vi "main.vi"() -> ()   [LabVIEW 2020]
uses:
  Libreria propria Chroma63204A/chr63204A_Error_conversion.vi
panel:
  out "CURR":dbl
  out "VOLT":dbl
  out "Numeric":i32
  out "element":dbl
  out "x = y?":bool
  out "error out (no error) 2":errorcluster
  in  "timestep (s)":u32=1
  in  "Load from file":bool
  in  "Load Profile path":path=path "C:/Users/thoma/Desktop/Nuova cartella/Load profile.csv"
  out "error out (no error)":errorcluster
  in  "Save path":path=path "C:/Users/thoma/Desktop/main/log.csv"
  in  "Stop Button":bool
  in  "LOAD":bool
  in  "Set current (A)":dbl
  in  "error in (no error)":errorcluster
  in  "Chroma USB port":refnum<visa-resource-name>
  in  "Mode":u16(ring)=1 items=["Z", "CC", "CR", "CV", "CP", "CCD", "CRD", "BAT", "SWD", "OCP", "CCS", "CZ", "CVCC", "CRCC", "CVCR", "AUTO", "PROG", "UDW", "EXT"]
  out "LOAD_STATE":bool
  out "Current imposed":dbl
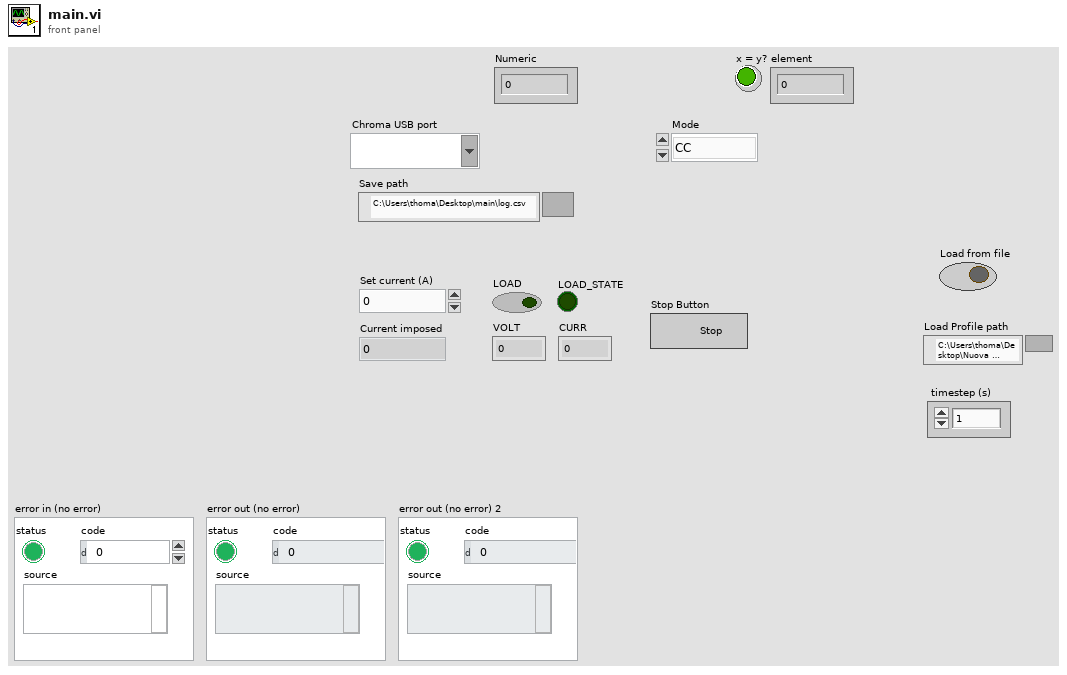
[diagram p1: front panel]
types:
  T1 = enum16{"open", "replace", "create", "open or create", "replace or create", "replace or create with confirmation"}
  T2 = enum8{"Enabled", "Disabled", "Disabled and Grayed Out"}
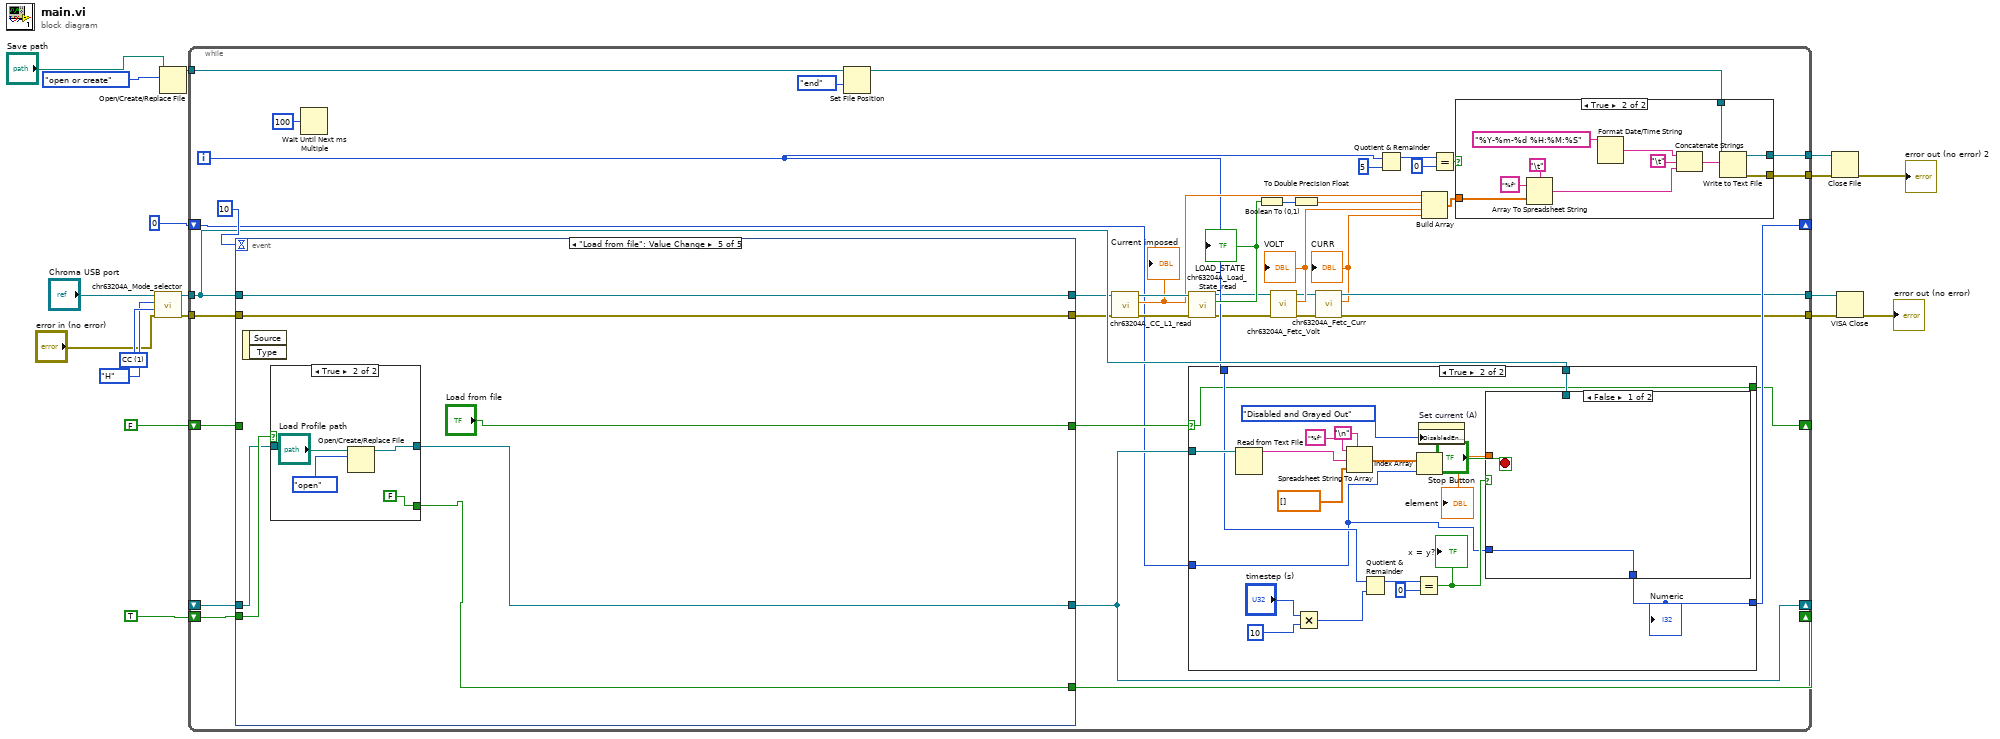
[diagram p0: block diagram]
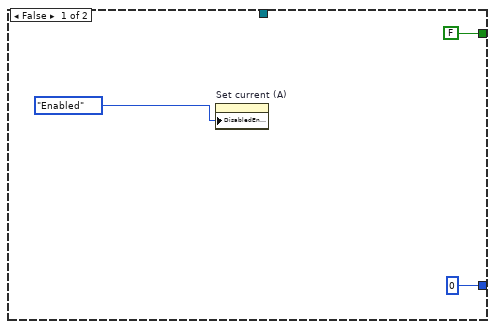
[diagram p2: hidden frame]
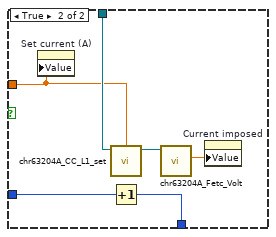
[diagram p3: hidden frame]
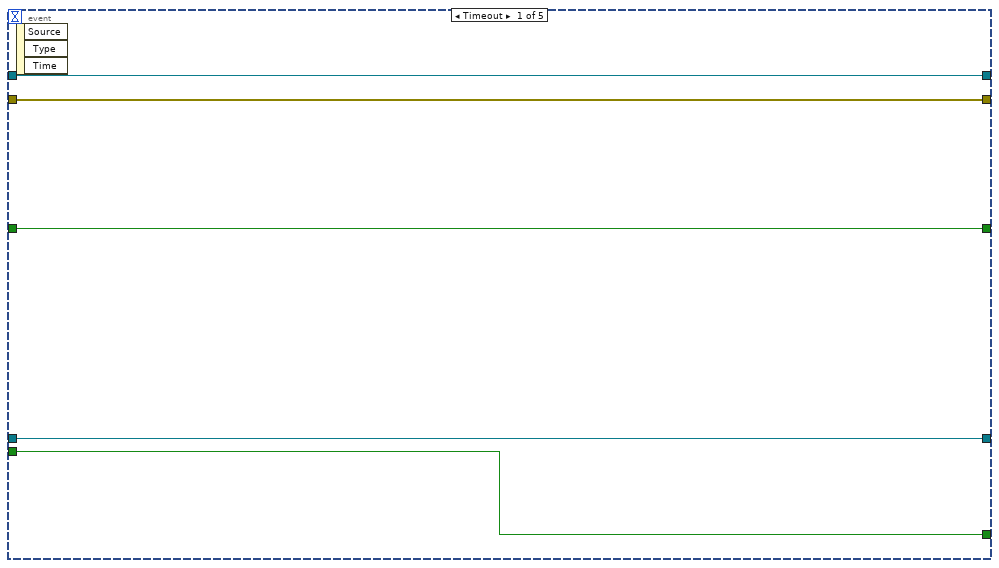
[diagram p5: hidden frame]
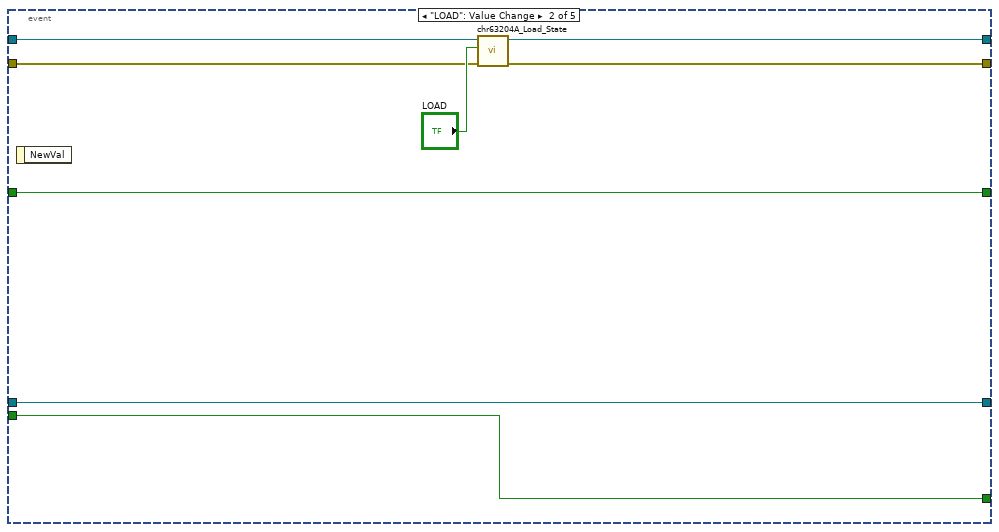
[diagram p6: hidden frame]
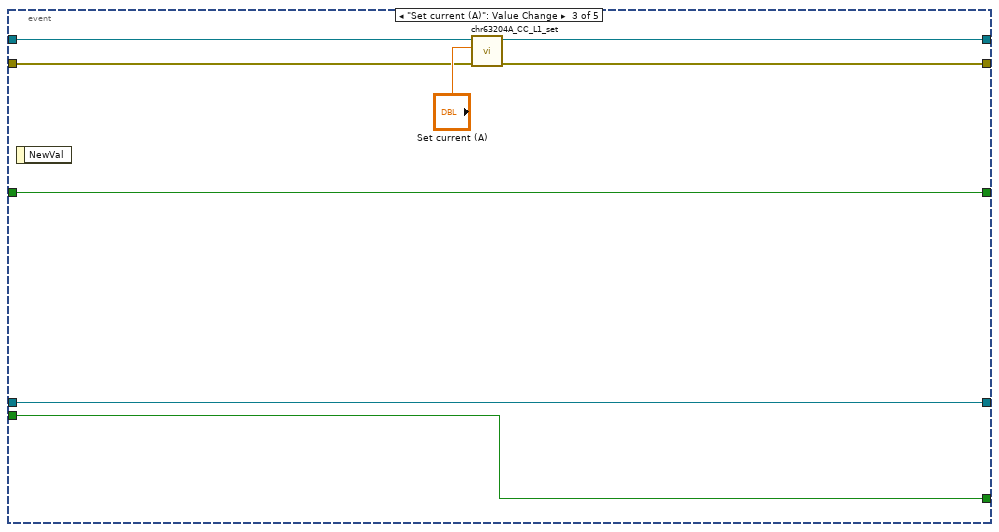
[diagram p7: hidden frame]
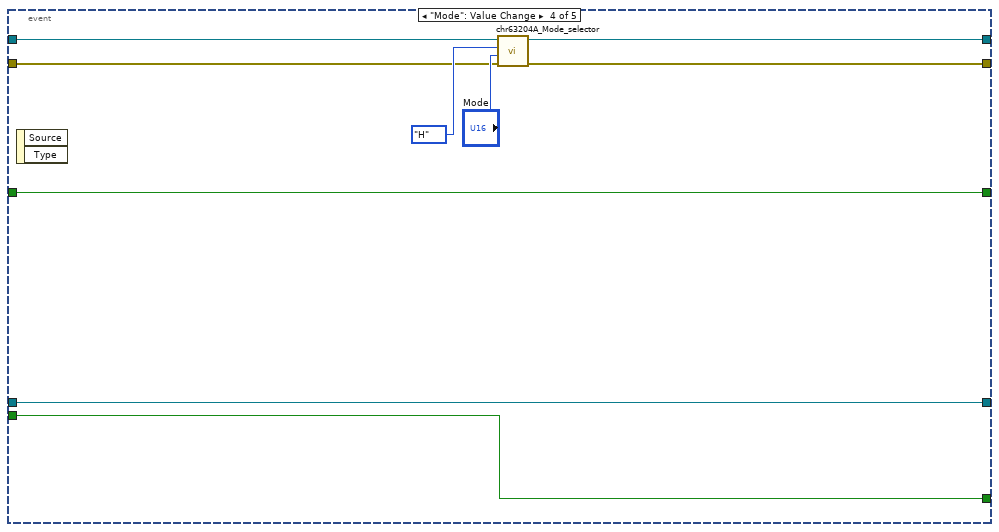
[diagram p8: hidden frame]
diagram:
  w17 = u16 1 items=["Z", "CC", "CR", "CV", "CP", "CCD", "CRD", "BAT", "SWD", "OCP", "CCS", "CZ", "CVCC", "CRCC", "CVCR", "AUTO", "PROG", "UDW", "EXT"] ("Mode 2")
  n1 = call "chr63204A_Mode_selector.vi"("error in (no error)"="error in (no error)", "Mode"=w17, "Level"=enum16{"Z", "L", "M", "H"}."H", "VISA resource name"="Chroma USB port") -> ("error out"=w13:errorcluster, "VISA resource name out"=w14:refnum<visa-resource-name>)  [unwired: 6 in]
  n2 = Open/Create/Replace File(file path (use dialog)="Save path", operation (0:open)=T1."open or create") -> (refnum out=w10:refnum<file>)  [unwired: 4 in, 2 out]
  n3 = while {
    tunnel: w14 -> [w58]
    tunnel: w13 -> [w57]
    tunnel: w10 -> [w50]
    tunnel: [w48] -> w9
    tunnel: [w47] -> w8
    tunnel: [w21] -> w7
    tunnel: [w20] -> w6
    shift-right: [w46] -> _
    shift-left: TRUE -> [w45]
    shift-right: [w31] -> _
    shift-left: _ -> [w44]
    shift-right: [w29] -> _
    shift-left: 0 -> [w30]
    shift-right: [w27] -> _
    shift-left: FALSE -> [w28]
    i -> [w33]
    stop <- "Stop Button" stop-if-true
    n4 = event shown="[4] \"Load from file\": Value Change" {
      selector: _ -> [_ _ _ _ _]
      dyn-events: _ -> [_ _ _ _ _]
      timeout: 10 -> [_ _ _ _ _]
      tunnel: w58 -> [w105 w112 w120 w128 w132]
      tunnel: w57 -> [w104 w111 w119 w127 w137]
      tunnel: [w105 w110 w118 w126 w132] -> w43
      tunnel: [w104 w109 w117 w125 w137] -> w42
      tunnel: [w103 w108 w116 w124 w135] -> w46
      tunnel: w45 -> [w103 w108 w116 w124 w136]
      tunnel: [w102 w107 w115 w123 w134] -> w31
      tunnel: w44 -> [w102 w107 w115 w123 w133]
      tunnel: [w101 w106 w114 w122 "Load from file"] -> w32
      tunnel: w28 -> [w101 w106 w114 w122 _]
      event Timeout {
        n5 = event-data() -> ()  [unwired: 1 in, 3 out]
      }
      event "LOAD": Value Change {
        n6 = event-data() -> ()  [unwired: 1 in, 1 out]
        n7 = call "chr63204A_Load_State.vi"("error in (no error)"=w111, "LOAD"="LOAD", "VISA resource name"=w112) -> ("error out"=w109:errorcluster, "VISA resource name out"=w110:refnum<visa-resource-name>)  [unwired: 7 in]
      }
      event "Set current (A)": Value Change {
        n8 = event-data() -> ()  [unwired: 1 in, 1 out]
        n9 = call "chr63204A_CC_L1_set.vi"("error in (no error)"=w119, "CC current"="Set current (A)", "VISA resource name"=w120) -> ("error out"=w117:errorcluster, "VISA resource name out"=w118:refnum<visa-resource-name>)  [unwired: 7 in]
      }
      event "Mode": Value Change {
        n10 = event-data() -> ()  [unwired: 1 in, 2 out]
        n11 = call "chr63204A_Mode_selector.vi"("error in (no error)"=w127, "Mode"="Mode", "Level"=enum16{"Z", "L", "M", "H"}."H", "VISA resource name"=w128) -> ("error out"=w125:errorcluster, "VISA resource name out"=w126:refnum<visa-resource-name>)  [unwired: 6 in]
      }
      event "Load from file": Value Change {
        n12 = event-data() -> ()  [unwired: 1 in, 2 out]
        n13 = case shown="True" w136 {
          selector: w136 -> [w139 _]
          tunnel: [w138 w141] -> w134
          tunnel: [w139 FALSE] -> w135
          tunnel: w133 -> [w138 _]
          frame False {
          }
          frame True {
            n14 = Open/Create/Replace File(file path (use dialog)="Load Profile path", operation (0:open)=T1."open") -> (refnum out=w141:refnum<file>)  [unwired: 4 in, 2 out]
          }
        }
      }
    }
    n15 = Wait Until Next ms Multiple(millisecond multiple=u32 100) -> ()  [unwired: 1 out]
    n16 = Set File Position(refnum=w50, from (0:start)=enum16{"start", "end", "current"}."end") -> (refnum out=w49:refnum<file>)  [unwired: 2 in, 1 out]
    n17 = call "chr63204A_CC_L1_read.vi"("error in (no error)"=w42, "VISA resource name"=w43) -> ("error out"=w40:errorcluster, "Value"=w39:dbl, "VISA resource name out"=w41:refnum<visa-resource-name>)  [unwired: 7 in]
    "Current imposed" <- w39
    n18 = call "chr63204A_Load_State_read.vi"("error in (no error)"=w40, "VISA resource name"=w41) -> ("error out"=w25:errorcluster, "LOAD_STATE"=w55:bool, "VISA resource name out"=w26:refnum<visa-resource-name>)  [unwired: 7 in]
    "LOAD_STATE" <- w55
    n19 = case shown="True" w32 {
      selector: w32 -> [_ w65]
      tunnel: w31 -> [_ w79]
      tunnel: w58 -> [_ w74]
      tunnel: w30 -> [_ w63]
      tunnel: w33 -> [_ w68]
      tunnel: [0 w64] -> w29
      tunnel: [FALSE w65] -> w27
      frame False {
        n20 = property on="Set current (A)" class="DigNum (strict)"("DisabledEnum"=T2."Enabled" ("Disabled")) -> ()  [unwired: 2 in, 2 out]
      }
      frame True {
        n21 = Read from Text File(file (use dialog)=w79) -> (text=w80:string)  [unwired: 3 in, 3 out]
        n22 = Multiply(x="timestep (s)", y=u32 10) -> (x*y=w66:u32)
        n23 = Spreadsheet String To Array(delimiter (Tab)="\n", format string="%f", spreadsheet string=w80, array type (2D Dbl)=dbl[] []) -> (array=w76:dbl[])
        n24 = Quotient & Remainder(x=w68, y=w66) -> (x-y*floor(x/y)=w70:u32)  [unwired: 1 out]
        n25 = Equal?(x=w70, y=0) -> (x = y?=w67:bool)
        "x = y?" <- w67
        n26 = Index Array(array=w76, index=w63) -> (element=w71:dbl)
        "element" <- w71
        n27 = property on="Set current (A)" class="DigNum (strict)"("DisabledEnum"=T2."Disabled and Grayed Out" ("Disabled")) -> ()  [unwired: 2 in, 2 out]
        n28 = case shown="False" w67 {
          tunnel: w74 -> [_ w88]
          tunnel: w71 -> [_ w85]
          tunnel: [w82 w83] -> w64
          tunnel: w63 -> [w82 w84]
          frame False {
          }
          frame True {
            n29 = property on="Set current (A)" class="DigNum (strict)"("Value"=w85) -> ()  [unwired: 2 in, 2 out]
            n30 = call "chr63204A_CC_L1_set.vi"("CC current"=w85, "VISA resource name"=w88) -> ("VISA resource name out"=w87:refnum<visa-resource-name>)  [unwired: 8 in, 1 out]
            n31 = Increment(x=w84) -> (x+1=w83:i32)
            n32 = call "chr63204A_Fetc_Volt.vi"("VISA resource name"=w87) -> ("Value"=w86:dbl)  [unwired: 8 in, 2 out]
            n33 = property on="Current imposed" class="DigNum (strict)"("Value"=w86) -> ()  [unwired: 2 in, 2 out]
          }
        }
        "Numeric" <- w64
      }
    }
    n34 = Boolean To (0,1)(Boolean=w55) -> (0, 1=w56:i16)
    n35 = call "chr63204A_Fetc_Volt.vi"("error in (no error)"=w25, "VISA resource name"=w26) -> ("error out"=w22:errorcluster, "Value"=w24:dbl, "VISA resource name out"=w23:refnum<visa-resource-name>)  [unwired: 7 in]
    "VOLT" <- w24
    n36 = To Double Precision Float(number=w56) -> (double precision float=w53:dbl)
    n37 = call "chr63204A_Fetc_Curr.vi"("error in (no error)"=w22, "VISA resource name"=w23) -> ("error out"=w20:errorcluster, "Value"=w19:dbl, "VISA resource name out"=w21:refnum<visa-resource-name>)  [unwired: 7 in]
    "CURR" <- w19
    n38 = Quotient & Remainder(x=w33, y=5) -> (x-y*floor(x/y)=w36:i32)  [unwired: 1 out]
    n39 = Build Array(w39, w53, w24, w19) -> (w52:dbl[])
    n40 = Equal?(x=w36, y=0) -> (x = y?=w34:bool)
    n41 = case shown="True" w34 {
      tunnel: w52 -> [_ w98]
      tunnel: w49 -> [w89 w92]
      tunnel: [w89 w91] -> w48
      tunnel: [_ w90] -> w47
      frame False {
      }
      frame True {
        n42 = Array To Spreadsheet String(delimiter (Tab)="\t", array=w98, 3:"%f" ("format string")) -> (spreadsheet string=w95:string)
        n43 = Format Date/Time String(time format string (%c)="%Y-%m-%d %H:%M:%S") -> (date/time string=w96:string)  [unwired: 2 in]
        n44 = Concatenate Strings(w96, "\t", w95) -> (w93:string)
        n45 = Write to Text File(file (use dialog)=w92, text=w93) -> (refnum out=w91:refnum<file>, error out=w90:errorcluster)  [unwired: 2 in, 1 out]
      }
    }
  }
  n46 = Close File(refnum=w9, error in=w8) -> (error out=→"error out (no error) 2":errorcluster)  [unwired: 1 out]
  n47 = VISA Close(VISA resource name=w7, error in (no error)=w6) -> (error out=→"error out (no error)":errorcluster)
